vi "Read Rank.vi"(8 "error in":errorcluster, 11 "SG 8GHz Path Group in":refnum<class "SG 8GHz Path Group.lvclass">) -> (0 "error out":errorcluster, 2 "Rank":dbl, 3 "SG 8GHz Path Group out":refnum<class "SG 8GHz Path Group.lvclass">)   [LabVIEW 2023, in "RFFixtureCharact.PXI.lvlib" / "SG 8GHz Path Group.lvclass"]
uses:
  SG 8GHz Path Group.lvclass
  SG 8GHz Path Group.lvclass/SG 8GHz Path Group.ctl
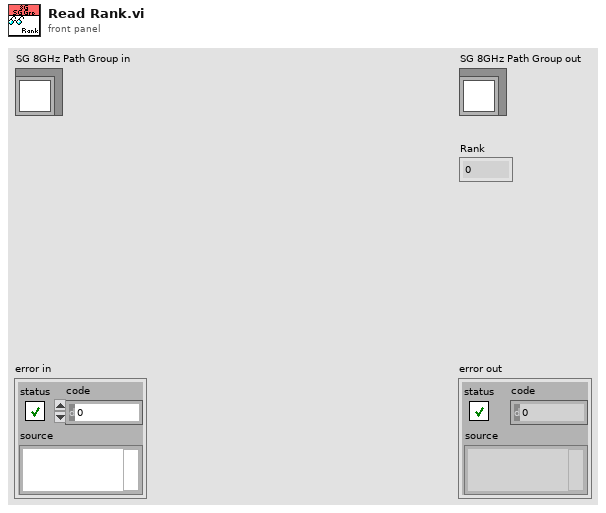
[diagram p1: front panel]
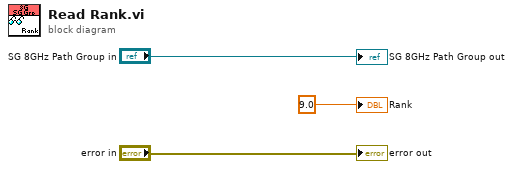
[diagram p0: block diagram]
diagram:
  "error out" <- "error in"
  "SG 8GHz Path Group out" <- "SG 8GHz Path Group in"
  "Rank" <- 9.0 ("Rank")
